vi "ELVIS III v1.0 RPC Session Map.vi"(8 "error in (no error)":errorcluster, 9 "Action":T2, 10 "Channel Names":string[](array[string]), 11 "Session":u32) -> (0 "error out":errorcluster, 3 "Session Infos":T1(array[cluster]))   [LabVIEW 2021]
uses:
  <vilib>/myRIO/Common/Instrument Driver Framework/ELVIS III v1.0/Resource Manager/typedefs/ELVIS III v1.0 RIO Session Map Action.ctl
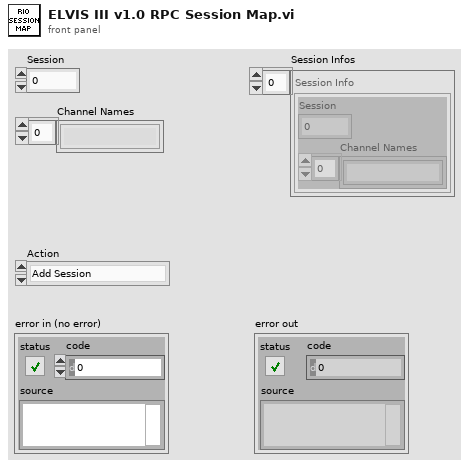
[diagram p1: front panel]
types:
  T1 = cluster{"Session":u32, "Channel Names":string[]}[]
  T2 = typedef "ELVIS III v1.0 RIO Session Map Action.ctl" = enum16{"Add Session", "Remove Session", "Get Active Sessions", "Get Owning Sessions"}
  T3 = enum32{"Bad", "Idle", "Run top level", "Running"}
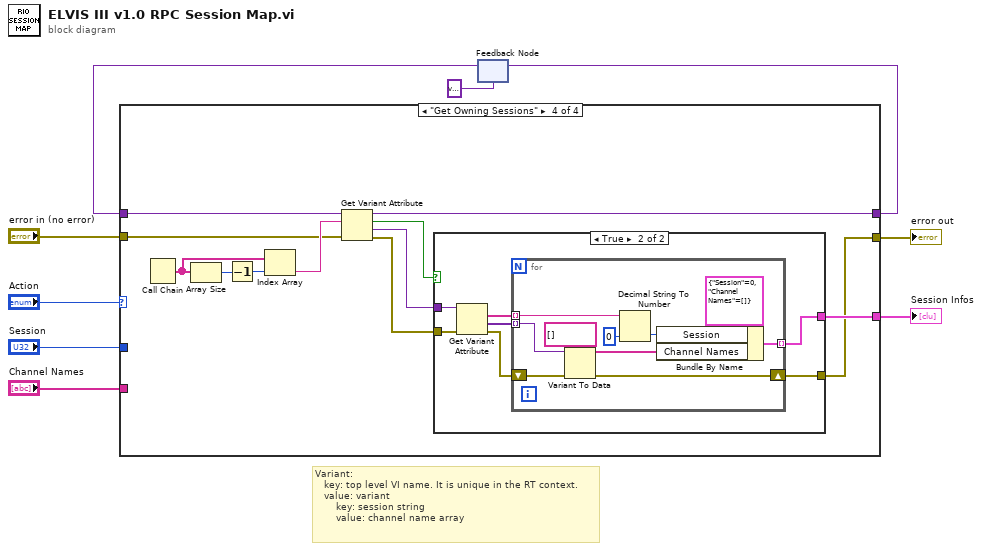
[diagram p0: block diagram]
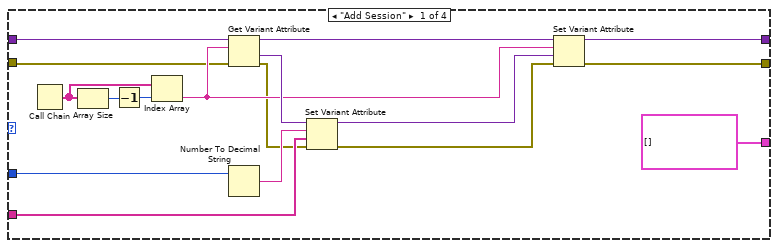
[diagram p2: hidden frame]
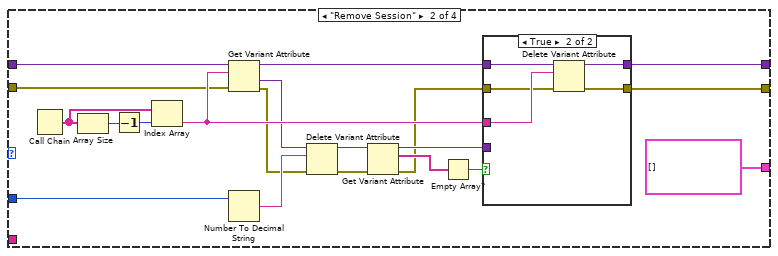
[diagram p3: hidden frame]
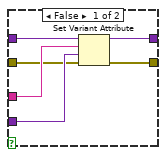
[diagram p4: hidden frame]
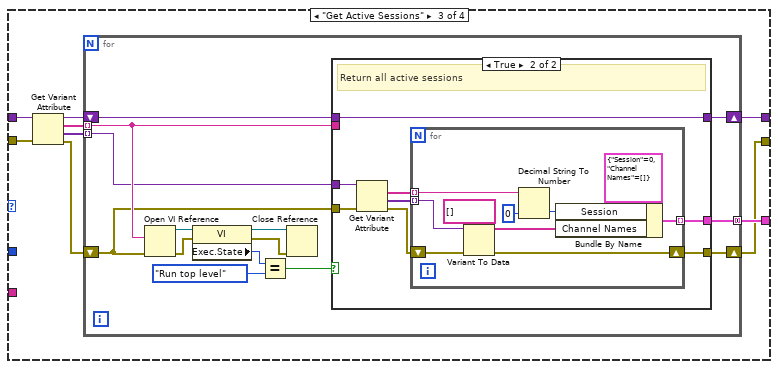
[diagram p5: hidden frame]
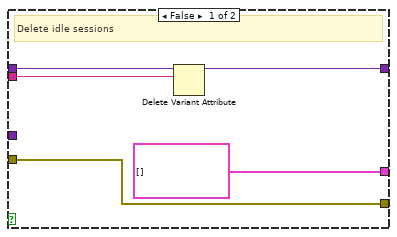
[diagram p6: hidden frame]
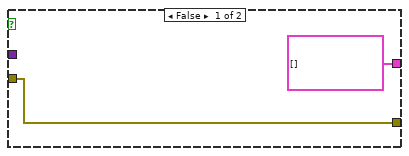
[diagram p7: hidden frame]
diagram:
  # "Variant:\n   key: top level VI name. It is unique in the RT context.\n   value: variant\n       key: session string\n       value: channel name array"
  n1 = feedback #1(variant) -> (w6:variant)
  n2 = case shown="\"Get Owning Sessions\"" "Action" {
    tunnel: "Channel Names" -> [w17 _ _ _]
    tunnel: [w21 w41 w62 w109] -> w7
    tunnel: w6 -> [w20 w46 w66 w111]
    tunnel: "Session" -> [w18 w38 _ _]
    tunnel: [T1 [] T1 [] w64 w106] -> w3
    tunnel: "error in (no error)" -> [w10 w31 w60 w110]
    tunnel: [w13 w27 w58 w105] -> w1
    frame "Add Session" {
      n3 = Call Chain() -> (call chain=w24:string[])
      n4 = Array Size(array=w24) -> (size(s)=w26:i32)
      n5 = Decrement(x=w26) -> (x-1=w25:i32)
      n6 = Index Array(array=w24, index=w25) -> (element=w22:string)
      n7 = Get Variant Attribute(Variant=w20, name=w22, error in=w10) -> (duplicate Variant=w19:variant, value=w23:variant, error out=w11:errorcluster)  [unwired: 1 in, 1 out]
      n8 = Number To Decimal String(number=w18) -> (decimal integer string=w16:string)  [unwired: 1 in]
      n9 = Set Variant Attribute(Variant=w23, name=w16, value=w17, error in=w11) -> (Variant out=w15:variant, error out=w12:errorcluster)  [unwired: 1 out]
      n10 = Set Variant Attribute(Variant=w19, name=w22, value=w15, error in=w12) -> (Variant out=w21:variant, error out=w13:errorcluster)  [unwired: 1 out]
    }
    frame "Remove Session" {
      n11 = Call Chain() -> (call chain=w43:string[])
      n12 = Array Size(array=w43) -> (size(s)=w45:i32)
      n13 = Decrement(x=w45) -> (x-1=w44:i32)
      n14 = Index Array(array=w43, index=w44) -> (element=w40:string)
      n15 = Get Variant Attribute(Variant=w46, name=w40, error in=w31) -> (duplicate Variant=w42:variant, value=w39:variant, error out=w30:errorcluster)  [unwired: 1 in, 1 out]
      n16 = Number To Decimal String(number=w38) -> (decimal integer string=w37:string)  [unwired: 1 in]
      n17 = Delete Variant Attribute(4:w30, 6:w37, 7:w39) -> (0:w29:errorcluster, 3:w36:variant)  [unwired: 1 out]
      n18 = Get Variant Attribute(Variant=w36, error in=w29) -> (duplicate Variant=w35:variant, names=w34:string[], error out=w28:errorcluster)  [unwired: 2 in, 1 out]
      n19 = Empty Array?(array=w34) -> (empty?=w33:bool)
      n20 = case shown="True" w33 {
        tunnel: w42 -> [w52 w57]
        tunnel: [w51 w56] -> w41
        tunnel: w40 -> [w50 w55]
        tunnel: w35 -> [w49 _]
        tunnel: w28 -> [w47 w54]
        tunnel: [w48 w53] -> w27
        frame False {
          n21 = Set Variant Attribute(Variant=w52, name=w50, value=w49, error in=w47) -> (Variant out=w51:variant, error out=w48:errorcluster)  [unwired: 1 out]
        }
        frame True {
          n22 = Delete Variant Attribute(4:w54, 6:w55, 7:w57) -> (0:w53:errorcluster, 3:w56:variant)  [unwired: 1 out]
        }
      }
    }
    frame "Get Active Sessions" {
      n23 = Get Variant Attribute(Variant=w66, error in=w60) -> (duplicate Variant=w63:variant, names=w65:string[], values=w61:variant[], error out=w59:errorcluster)  [unwired: 2 in]
      n24 = for {
        tunnel: w65 -> [w71] mode=indexing
        tunnel: [w69] -> w64 mode=concatenating
        shift-right: [w73] -> w62
        shift-left: w63 -> [w72]
        tunnel: w61 -> [w70] mode=indexing
        shift-right: [w67] -> w58
        shift-left: w59 -> [w68]
        n25 = Open VI Reference(vi path=w71, error in (no error)=w68) -> (vi reference=w80:refnum<vi>, error out=w75:errorcluster)  [unwired: 4 in]
        n26 = property class="VI"(reference=w80, error in=w75) -> (reference out=w77:refnum<vi>, error out=w76:errorcluster, "Exec.State"=w79:T3)
        n27 = Equal?(x=w79, y=T3."Run top level" ("Execution:State")) -> (x = y?=w74:bool)
        n28 = Close Reference(reference=w77, error in (no error)=w76) -> ()  [unwired: 1 out]
        n29 = case shown="True" w74 {
          tunnel: [w84 w93] -> w73
          tunnel: w72 -> [w85 w93]
          tunnel: w71 -> [w83 _]
          tunnel: w70 -> [_ w92]
          tunnel: [T1 [] w89] -> w69
          tunnel: w68 -> [w81 w88]
          tunnel: [w81 w86] -> w67
          frame False {
            # "Delete idle sessions"
            n30 = Delete Variant Attribute(6:w83, 7:w85) -> (3:w84:variant)  [unwired: 1 in, 2 out]
          }
          frame True {
            # "Return all active sessions"
            n31 = Get Variant Attribute(Variant=w92, error in=w88) -> (names=w91:string[], values=w90:variant[], error out=w87:errorcluster)  [unwired: 2 in, 1 out]
            n32 = for {
              tunnel: w91 -> [w103] mode=indexing
              tunnel: w90 -> [w96] mode=indexing
              tunnel: [w98] -> w89 mode=indexing
              shift-right: [w94] -> w86
              shift-left: w87 -> [w95]
              n33 = Variant To Data(error in=w95, type=string[] [] ("Channel Names"), Variant=w96) -> (data=w101:string[], error out=w94:errorcluster)
              n34 = Decimal String To Number(string=w103, default (0L)=u32 0 ("default (0 I32)")) -> (number=w99:u32)  [unwired: 1 in, 1 out]
              n35 = Bundle By Name(cluster=cluster{"Session":u32, "Channel Names":string[]} {"Session"=0, "Channel Names"=[]} ("Session Info"), "Session"=w99, "Channel Names"=w101) -> (w98:cluster{"Session":u32, "Channel Names":string[]})
            }
          }
        }
      }
    }
    frame "Get Owning Sessions" {
      n36 = Call Chain() -> (call chain=w114:string[])
      n37 = Array Size(array=w114) -> (size(s)=w112:i32)
      n38 = Decrement(x=w112) -> (x-1=w113:i32)
      n39 = Index Array(array=w114, index=w113) -> (element=w115:string)
      n40 = Get Variant Attribute(Variant=w111, name=w115, error in=w110) -> (duplicate Variant=w109:variant, found=w104:bool, value=w108:variant, error out=w107:errorcluster)  [unwired: 1 in]
      n41 = case shown="True" w104 {
        tunnel: w108 -> [_ w121]
        tunnel: w107 -> [w117 w120]
        tunnel: [T1 [] w119] -> w106
        tunnel: [w117 w118] -> w105
        frame False {
        }
        frame True {
          n42 = Get Variant Attribute(Variant=w121, error in=w120) -> (names=w124:string[], values=w123:variant[], error out=w122:errorcluster)  [unwired: 2 in, 1 out]
          n43 = for {
            tunnel: w124 -> [w134] mode=indexing
            tunnel: w123 -> [w127] mode=indexing
            tunnel: [w129] -> w119 mode=indexing
            shift-right: [w125] -> w118
            shift-left: w122 -> [w126]
            n44 = Variant To Data(error in=w126, type=string[] [] ("Channel Names"), Variant=w127) -> (data=w132:string[], error out=w125:errorcluster)
            n45 = Decimal String To Number(string=w134, default (0L)=u32 0 ("default (0 I32)")) -> (number=w130:u32)  [unwired: 1 in, 1 out]
            n46 = Bundle By Name(cluster=cluster{"Session":u32, "Channel Names":string[]} {"Session"=0, "Channel Names"=[]} ("Session Info"), "Session"=w130, "Channel Names"=w132) -> (w129:cluster{"Session":u32, "Channel Names":string[]})
          }
        }
      }
    }
  }
  "Session Infos" <- w3
  "error out" <- w1
  n47 = feedback-in #1(w7) -> ()
